vi "LowLevelError.vi"() -> ()   [LabVIEW 2019]
panel:
  in  "Low Level Error":errorcluster
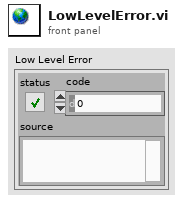
[diagram p1: front panel]
diagram:
